vi "le_escreve_digital.vi"() -> ()   [LabVIEW 2020]
uses:
  <vilib>/DAQmx/write.llb/DAQmx Write (Digital Bool 1Line 1Point).vi
  <vilib>/DAQmx/read.llb/DAQmx Read (Digital Bool 1Line 1Point).vi
  <vilib>/DAQmx/create/channels.llb/DAQmx Create Channel (DO-Digital Output).vi
  <vilib>/DAQmx/create/channels.llb/DAQmx Create Channel (DI-Digital Input).vi
  <vilib>/DAQmx/miscellaneous.llb/DAQmx Fill In Error Info.vi
panel:
  out "data 2":bool
  in  "task in 2":refnum<k21>
  in  "lines 2":tag
  out "error out 2":errorcluster
  in  "task in":refnum<k21>
  in  "lines":tag
  in  "data":bool
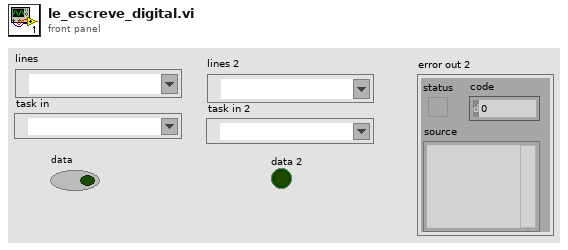
[diagram p1: front panel]
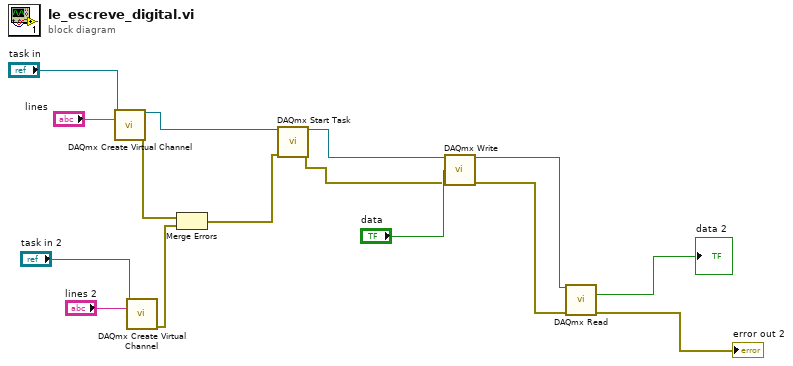
[diagram p0: block diagram]
diagram:
  n1 = call-poly <vilib>:"DAQmx Create Virtual Channel.vi"("task in"="task in", "lines"="lines") -> ("task out"=w15:refnum<k21>, "error out"=w4:errorcluster)  [unwired: 12 in]
  n2 = call-poly <vilib>:"DAQmx Create Virtual Channel.vi"("task in"="task in 2", "lines"="lines 2") -> ("error out"=w5:errorcluster)  [unwired: 12 in, 1 out]
  n3 = Merge Errors(w4, w5) -> (w3:errorcluster)
  n4 = call <vilib>:"DAQmx Start Task.vi"("task/channels in"=w15, "error in"=w3) -> ("task out"=w14:refnum<k21>, "error out"=w6:errorcluster)  [unwired: 12 in]
  n5 = call-poly <vilib>:"DAQmx Write.vi"("task/channels in"=w14, "data"="data", "error in"=w6) -> ("task out"=w2:refnum<k21>, "error out"=w1:errorcluster)  [unwired: 10 in, 1 out]
  n6 = call-poly <vilib>:"DAQmx Read.vi"("task/channels in"=w2, "error in"=w1) -> ("data"=→"data 2":bool, "error out"=→"error out 2":errorcluster)  [unwired: 11 in, 1 out]
